vi "MEMR-Initialize Hardware.vi"(5 "Params":T31, 11 "error in (no error)":errorcluster) -> (8 "AO":T1 {"noiseChan"."Filter"."Stages"."IIR Filter"."Forward Coefficients" format="%.4f"; "noiseChan"."Filter"."Stages"."IIR Filter"."Reverse Coefficients" format="%.4f"}, 15 "error out":errorcluster)   [LabVIEW 2020]
uses:
  Typedefs/MEMR-Params.ctl
  Typedefs/MEMR-Probe.ctl
  Typedefs/MEMR-Elicitor.ctl
  Human Studies/SFM Frontend/LV Source/Typedefs/HSTS-Transducer.ctl
  Typedefs/MEMR-Sequence.ctl
  Typedefs/MEMR-Analysis.ctl
  Typedefs/MEMR-Timing.ctl
  Typedefs/MEMR-AO Data.ctl
  Signal Synthesis VIs/3rd Generation/XControls/Stimulus Channel (G3)/Full Stimulus Channel Data.ctl
  Signal Synthesis VIs/3rd Generation/XControls/Waveform XControls/Waveform (G3)/Waveform Data.ctl
  Signal Synthesis VIs/3rd Generation/Waveform VIs/Waveform Enum (V3).ctl
  Signal Synthesis VIs/3rd Generation/XControls/Waveform XControls/Tone (G3)/Tone.Properties.ctl
  Signal Synthesis VIs/Waveform VIs/Pulse Train VIs/Pulse Train Params.ctl
  Signal Synthesis VIs/Waveform VIs/Pulse Train VIs/Pulse Polarity.ctl
  Signal Synthesis VIs/Waveform VIs/Pulse Train VIs/PT-Continuous State.ctl
  Signal Synthesis VIs/3rd Generation/Waveform VIs/Noise VIs/Noise (G3).ctl
  Signal Synthesis VIs/3rd Generation/Waveform VIs/Noise VIs/Noise (G3).Properties.ctl
  Signal Synthesis VIs/3rd Generation/Waveform VIs/Noise VIs/Noise (G3).Data.ctl
  Signal Synthesis VIs/Waveform VIs/File VIs/StimFile-Params.ctl
  Signal Synthesis VIs/Waveform VIs/FM Sweep VIs/FM Sweep Params.ctl
  Signal Synthesis VIs/Waveform VIs/Chirp Train VIs/Chirp Train.ctl
  Signal Synthesis VIs/Waveform VIs/Chirp Train VIs/Chirp Train Params.ctl
  Signal Synthesis VIs/Waveform VIs/Complex Tone VIs/CT-Params.ctl
  Signal Synthesis VIs/Waveform VIs/Complex Tone VIs/CT-Phase Enum.ctl
  Signal Synthesis VIs/Waveform VIs/Complex Tone VIs/CT-Runtime Data.ctl
  Signal Synthesis VIs/3rd Generation/XControls/Waveform XControls/FM Tone/Data.ctl
  Signal Synthesis VIs/3rd Generation/XControls/Waveform XControls/Vowel/Vowel.Properties.ctl
  Signal Synthesis VIs/3rd Generation/Waveform VIs/Ramp VIs/Ramp.Properties.ctl
  Signal Synthesis VIs/3rd Generation/XControls/Filter (G3)/Filter Data.ctl
  Signal Synthesis VIs/3rd Generation/XControls/Filter (G3)/Filter Type.ctl
  Signal Synthesis VIs/Filter VIs/Filter-Bandwidth Units.ctl
  Signal Synthesis VIs/Controls/Burst XCtl/Burst Data.ctl
  Signal Synthesis VIs/3rd Generation/XControls/Level (G3)/Level Data.ctl
  Signal Synthesis VIs/3rd Generation/XControls/Level (G3)/Level Units (G3).ctl
  Signal Synthesis VIs/3rd Generation/XControls/Advanced Options (G3)/Advanced Options (G3).ctl
  Signal Synthesis VIs/Modulation VIs/SAM VIs/SAM Params.ctl
  Signal Synthesis VIs/3rd Generation/Typedefs/Destination.ctl
  Signal Synthesis VIs/3rd Generation/XControls/Filter (G3)/Filter (G3).xctl
  Signal Synthesis VIs/3rd Generation/XControls/Level (G3)/Level (G3).xctl
  Signal Synthesis VIs/Controls/Burst XCtl/Burst Control.xctl
  Signal Synthesis VIs/3rd Generation/XControls/Waveform XControls/Tone (G3)/Tone (G3).xctl
  Signal Synthesis VIs/3rd Generation/XControls/Waveform XControls/FM Tone/FM Tone.xctl
  Signal Synthesis VIs/3rd Generation/XControls/Waveform XControls/Vowel/Vowel.xctl
  Signal Synthesis VIs/3rd Generation/XControls/Waveform XControls/Waveform (G3)/Waveform (G3).xctl
  Signal Synthesis VIs/3rd Generation/XControls/Advanced Options (G3)/Advanced Options (G3).xctl
  Signal Synthesis VIs/3rd Generation/XControls/Stimulus Channel (G3)/Stimulus Channel (G3).xctl
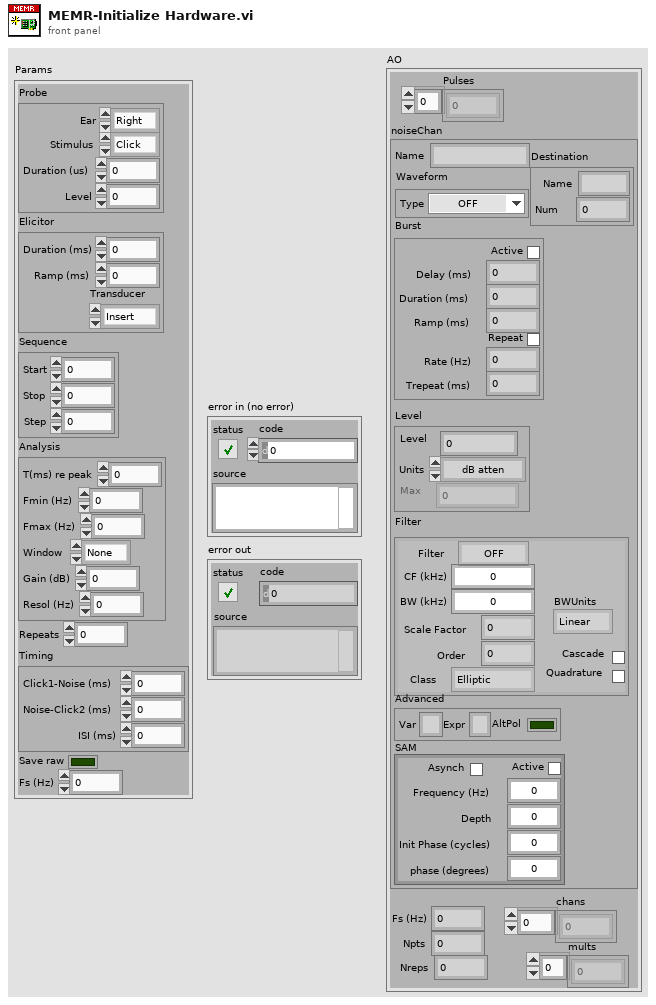
[diagram p1: front panel]
types:
  T1 = typedef "MEMR-AO Data.ctl" = cluster{"Pulses":dbl[], "noiseChan":T2, "Fs (Hz)":dbl, "Npts":i32, "mults":dbl[], "chans":i32[], "Nreps":i32}
  T2 = typedef "Stimulus Channel (G3).xctl/Full Stimulus Channel Data.ctl" = cluster{"Waveform":T3, "Filter":T22, "Burst":T25, "Level":T26, "Name":string, "Advanced":T28, "SAM":T29, "Destination":T30}
  T3 = typedef "Waveform (G3).xctl/Waveform Data.ctl" = cluster{"Type":T4, "Tone":T5, "Pulse Train":T6, "Noise":T9, "File":T12, "FMSweep":T13, "Chirp Train":T14, "Complex Tone":cluster{"Params":T16, "Data":T18}, "FM":T19, "Vowel":T20, "Ramp":T21}
  T4 = typedef "Waveform Enum (V3).ctl" = enum16{"OFF", "Tone", "Noise", "Pulse Train", "File", "FM Sweep", "Chirp Train", "Complex Tone", "FM Tone", "Vowel", "Ramp"}
  T5 = typedef "Tone (G3).xctl/Tone.Properties.ctl" = cluster{"Frequency (kHz)":dbl, "Phase (cycles)":dbl, "Random phase":bool}
  T6 = typedef "Pulse Train Params.ctl" = cluster{"Pulse width (us)":dbl, "Pulse rate (Hz)":dbl, "Gap (ms)":dbl, "Polarity":T7, "PT State":T8, "Asynch":bool}
  T7 = typedef "Pulse Polarity.ctl" = enum16{"POS", "NEG", "POS-NEG", "NEG-POS"}
  T8 = typedef "PT-Continuous State.ctl" = cluster{"Template":dbl[], "Nperiod":i32, "Index":i32, "Pulse Rate (Hz)":dbl, "Phase (cycles)":dbl, "Noff":i32}
  T9 = typedef "Noise (G3).ctl" = cluster{"Properties":T10, "Data":T11}
  T10 = typedef "Noise (G3).Properties.ctl" = cluster{"InvFilt":bool, "Aweight":bool, "Seed":i32, "Tokens":i32, "Brickwall":bool}
  T11 = typedef "Noise (G3).Data.ctl" = cluster{"TokenNum":i32}
  T12 = typedef "StimFile-Params.ctl" = cluster{"Filename":path, "Signal":dbl[], "Channel":i32, "stream":bool, "offset":i32, "nreps":i32, "loops":i32, "Randomize":bool, "order":i32[], "Seed":i32, "Tokens":i32}
  T13 = typedef "FM Sweep Params.ctl" = cluster{"Rate (oct/s)":dbl, "Fmin (Hz)":dbl, "Fmax (Hz)":dbl, "Ramp (ms)":dbl, "Linear":bool}
  T14 = typedef "Chirp Train.ctl" = cluster{"Params":T15, "Data":cluster{"WF":dbl[]}}
  T15 = typedef "Chirp Train Params.ctl" = cluster{"Fmin (kHz)":dbl, "Fmax (kHz)":dbl, "Compensate":bool, "Duration (ms)":dbl}
  T16 = typedef "CT-Params.ctl" = cluster{"F0 (Hz)":dbl, "Band":cluster{"Flow (Hz)":dbl, "Fhigh (Hz)":dbl}, "Phase":T17, "Min F0 (Hz)":dbl, "Max F0 (Hz)":dbl, "ContinRandPhase":bool, "Max peak factor":dbl, "Max mod depth":dbl, "MinHarmNum":i32, "MaxHarmNum":i32, "Level Mode":enum16{"per component", "overall rms"}, "% jitter":dbl}
  T17 = typedef "CT-Phase Enum.ctl" = enum16{"Cosine", "Random", "Alternating"}
  T18 = typedef "CT-Runtime Data.ctl" = cluster{"Ncomp":i32, "MinHarm":i32, "Phase":dbl[], "Amplitude":dbl[], "Npts/frame":i32, "Last F0":dbl, "Fmin":dbl, "Fmax":dbl, "Lslope":dbl, "randphase":bool, "overall rms":bool, "fmult":dbl[], "jittered":bool}
  T19 = typedef "FM Tone.xctl/Data.ctl" = cluster{"Carrier (kHz)":dbl, "ModRate (Hz)":dbl, "Depth (Hz)":dbl, "Phase (cycles)":dbl}
  T20 = typedef "Vowel.xctl/Vowel.Properties.ctl" = cluster{"Freqs":string, "Set level":enum16{"Total", "Per component"}, "Freq":dbl[], "weights":dbl[]}
  T21 = typedef "Ramp.Properties.ctl" = cluster{"Duration (ms)":dbl}
  T22 = typedef "Filter (G3).xctl/Filter Data.ctl" = cluster{"Type":T23, "CF (kHz)":dbl, "BW (kHz)":dbl, "Cascade":bool, "Quadrature":bool, "Scale Factor":dbl, "Stages":cluster{"IIR Filter":cluster{"filter structure":enum32{"IIR 2nd Order", "IIR 4th Order"}, "Reverse Coefficients":dbl[], "Forward Coefficients":dbl[]}, "State":dbl[]}[], "Class":enum16{"Elliptic", "Butterworth"}, "Order":i32, "BWUnits":T24}
  T23 = typedef "Filter (G3).xctl/Filter Type.ctl" = enum16{"OFF", "Lowpass", "Highpass", "Bandpass", "Bandstop"}
  T24 = typedef "Filter-Bandwidth Units.ctl" = enum16{"Linear", "Octaves", "Min-Max"}
  T25 = typedef "Burst Control.xctl/Burst Data.ctl" = cluster{"Active":bool, "Delay (ms)":dbl, "Duration (ms)":dbl, "Ramp (ms)":dbl, "Rate (Hz)":dbl, "Trepeat (ms)":dbl, "Repeat":bool}
  T26 = typedef "Level (G3).xctl/Level Data.ctl" = cluster{"Level":dbl, "Units":T27, "Max":dbl, "Data":cluster{"Multiplier":dbl, "Cal File":path, "Cal":cluster{"Freq (Hz)":dbl[], "Mag (dB SPL)":dbl[], "Phase (deg)":dbl[]}, "audiogram":path}}
  T27 = typedef "Level (G3).xctl/Level Units (G3).ctl" = enum16{"dB atten", "dB SPL", "dB re 1 Vrms", "dB V/Hz½", "mW", "dB HL", "Volts", "dB mW"}
  T28 = typedef "Advanced Options (G3).xctl/Advanced Options (G3).ctl" = cluster{"AltPol":bool, "Var":string, "Expr":string}
  T29 = typedef "SAM Params.ctl" = cluster{"Active":bool, "Frequency (Hz)":dbl, "Depth":dbl, "Init Phase (cycles)":dbl, "phase (degrees)":dbl, "Asynch":bool}
  T30 = typedef "Destination.ctl" = cluster{"Name":string, "Num":i32}
  T31 = typedef "MEMR-Params.ctl" = cluster{"Probe":T32, "Elicitor":T33, "Sequence":T35, "Analysis":T36, "Repeats":i32, "Timing":T37, "Save raw":bool, "Fs (Hz)":dbl}
  T32 = typedef "MEMR-Probe.ctl" = cluster{"Ear":enum16{"Right", "Left"}, "Stimulus":enum16{"Click", "Chirp"}, "Duration (us)":dbl, "Level":dbl}
  T33 = typedef "MEMR-Elicitor.ctl" = cluster{"Duration (ms)":dbl, "Ramp (ms)":dbl, "Transducer":T34}
  T34 = typedef "HSTS-Transducer.ctl" = enum16{"Insert", "TDH-39", "HD300", "ER-10X"}
  T35 = typedef "MEMR-Sequence.ctl" = cluster{"Start":dbl, "Stop":dbl, "Step":dbl}
  T36 = typedef "MEMR-Analysis.ctl" = cluster{"T(ms) re peak":dbl, "Fmin (Hz)":dbl, "Fmax (Hz)":dbl, "Window":enum16{"None", "Hanning", "Hamming"}, "Gain (dB)":dbl, "Resol (Hz)":dbl}
  T37 = typedef "MEMR-Timing.ctl" = cluster{"Click1-Noise (ms)":dbl, "Noise-Click2 (ms)":dbl, "ISI (ms)":dbl}
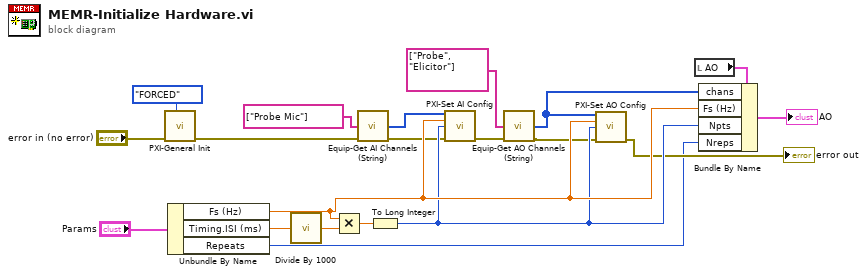
[diagram p0: block diagram]
diagram:
  n1 = call "PXI-General Init.vi"("Double Buffer Mode"=enum32{"OFF", "ENABLED", "FORCED"}."FORCED", "error in (no error)"="error in (no error)") -> ("error out"=w8:errorcluster)  [unwired: 9 in]
  n2 = Unbundle By Name("Params") -> ("Fs (Hz)"=w13:dbl, "Timing.ISI (ms)"=w18:dbl, "Repeats"=w9:i32)
  n3 = call "Divide By 1000.vi"("X"=w18) -> ("X/1000"=w17:dbl)
  n4 = Multiply(x=w13, y=w17) -> (x*y=w16:dbl)
  n5 = call "Equip-Get AI Channels (String).vi"("Inputs"=string[] ["Probe Mic"], "error in (no error)"=w8) -> ("AI Channels"=w6:i32[], "error out"=w7:errorcluster)  [unwired: 12 in]
  n6 = To Long Integer(number=w16) -> (32bit integer=w12:i32)
  n7 = call "PXI-Set AI Config.vi"("AI Channels"=w6, "Sampling Rate (Hz)"=w13, "Buffer Size"=w12, "error in (no error)"=w7) -> ("error out"=w4:errorcluster)  [unwired: 11 in]
  n8 = call "Equip-Get AO Channels (String).vi"("Channel Names"=string[] ["Probe", "Elicitor"], "error in (no error)"=w4) -> ("AO Channels"=w2:i32[], "error out"=w3:errorcluster)  [unwired: 12 in]
  n9 = call "PXI-Set AO Config.vi"("AO Channels"=w2, "Sampling Rate (Hz)"=w13, "Buffer Size"=w12, "error in (no error)"=w3) -> ("error out"=→"error out":errorcluster)  [unwired: 11 in]
  n10 = local read "AO"() -> (w14:T1)
  n11 = Bundle By Name(cluster=w14, "chans"=w2, "Fs (Hz)"=w13, "Npts"=w12, "Nreps"=w9) -> (→"AO":T1)
